vi "ReadTangoTestDoubleAttributes.vi"() -> ()   [LabVIEW 2009]
uses:
  tango_lv8/tango_vi.llb/ReadDoubleScalarAttribute.vi
  tango_lv8/tango_vi.llb/ReadDoubleSpectrumAttribute.vi
  tango_lv8/tango_vi.llb/ReadDoubleImageAttribute.vi
panel:
  out "Read/s":dbl
  out "Read/s":dbl
  in  "?":bool=TRUE
  in  "?":bool=TRUE
  out "Read/s":dbl
  in  "?":bool=TRUE
  out "error stack":string[](array[string])=["no error", "no error", "no error", "read_attributes"]
  out "error stack":string[](array[string])=["no error", "no error", "no error", "read_attributes"]
  out "error stack":string[](array[string])=["no error", "no error", "no error", "read_attributes"]
  out "scalar attr. value":dbl(graph)=99.87794428970838
  out "scalar attr. write value":dbl
  out "scalar attr. read value":dbl
  out "?":bool
  in  "attr_name":string="double_scalar"
  out "?":bool
  in  "attr_name":string="double_spectrum_ro"
  out "?":bool
  out "image attr. value":dbl[][](graph)
  out "spectrum attr. value":dbl[](graph)
  in  "attr_name":string="double_image_ro"
  in  "dev_name":string="tango/tangotest/1"
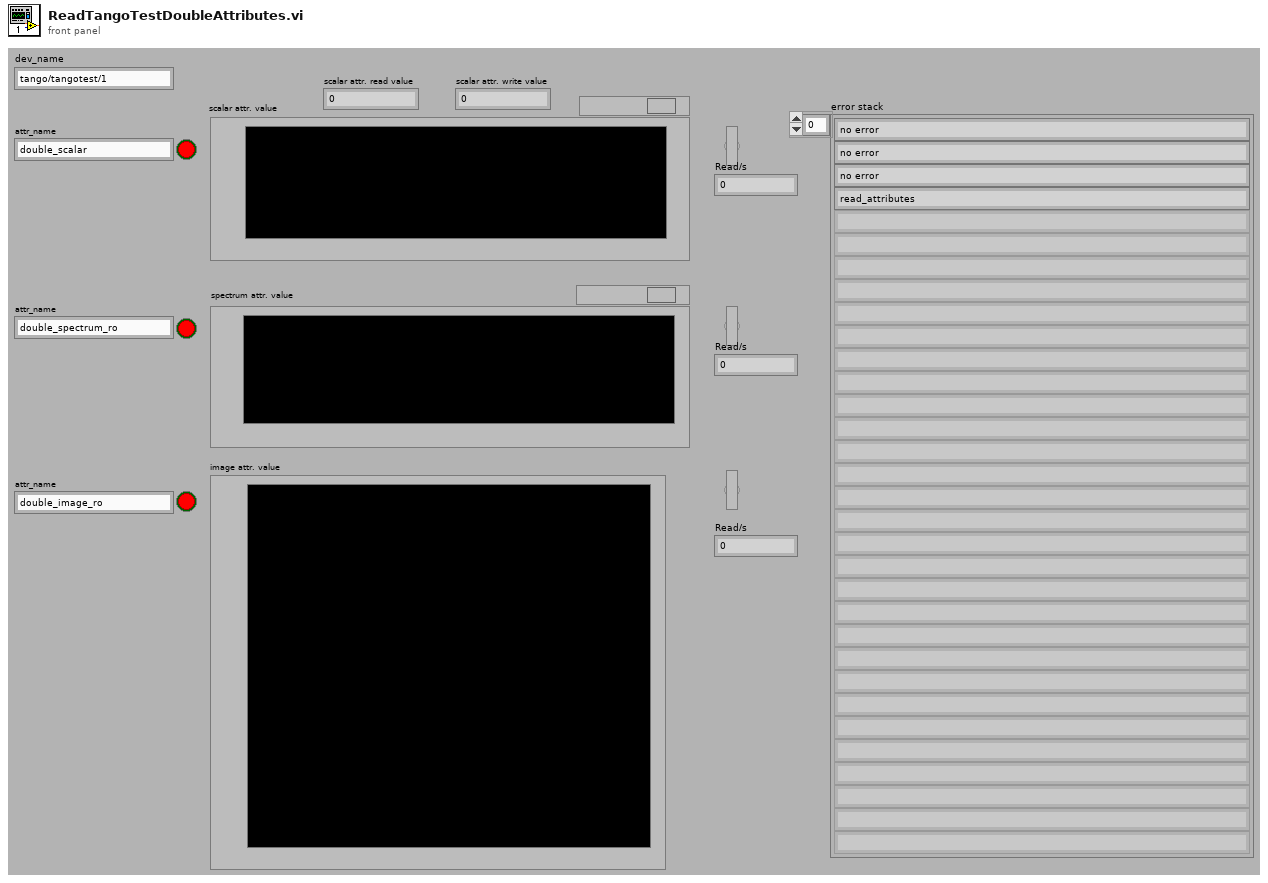
[diagram p1: front panel]
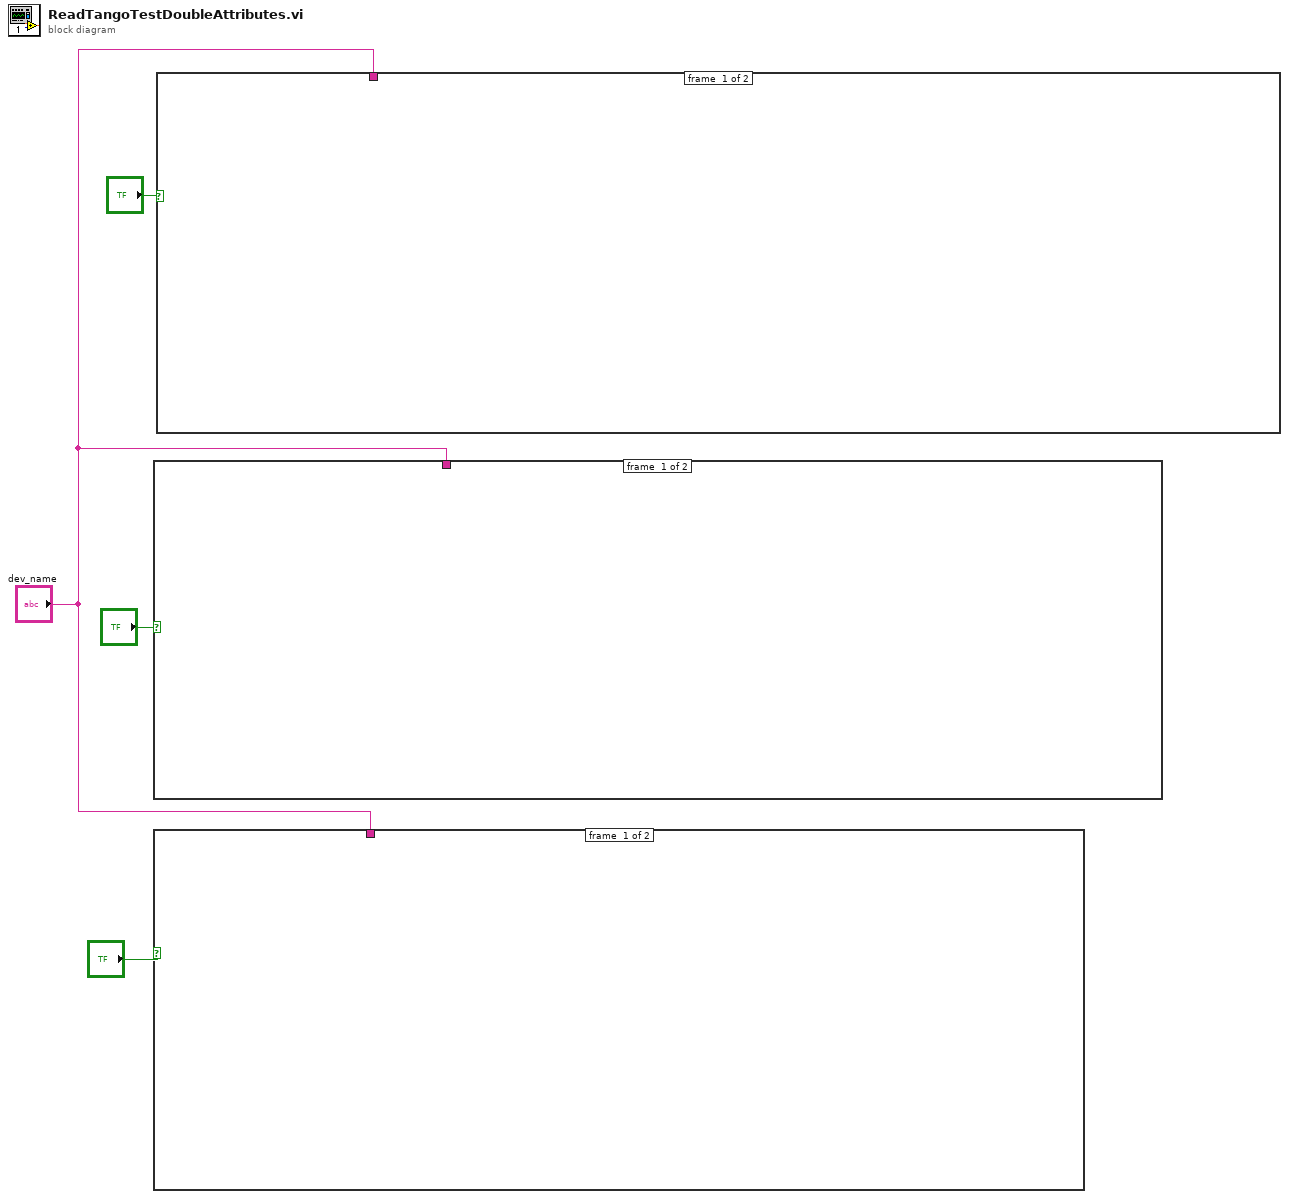
[diagram p0: block diagram]
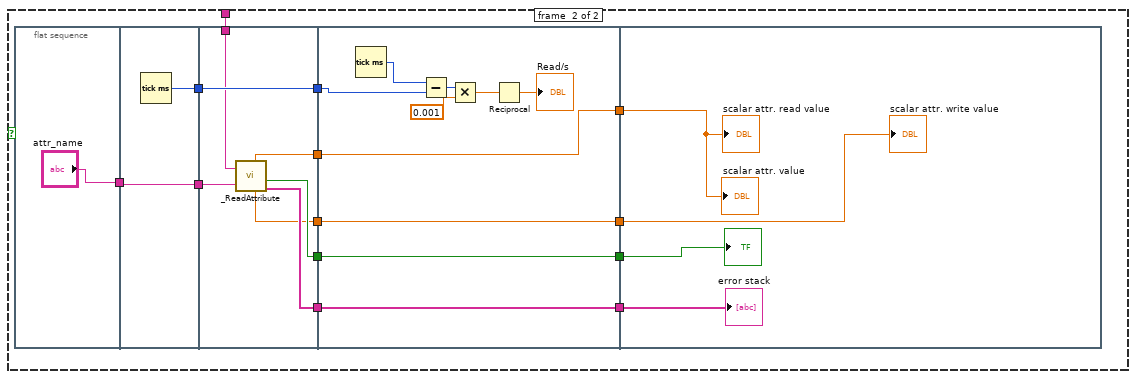
[diagram p2: hidden frame]
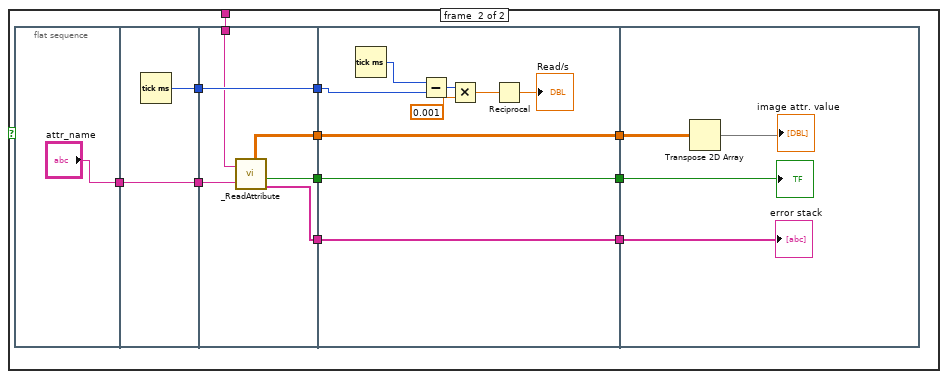
[diagram p3: hidden frame]
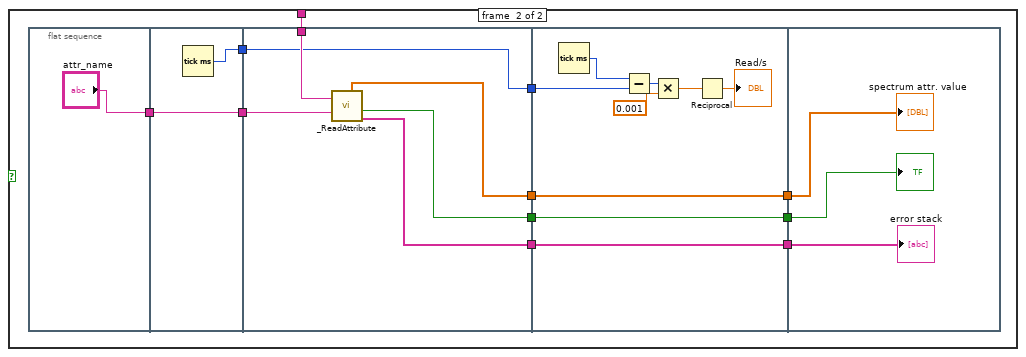
[diagram p4: hidden frame]
diagram:
  n1 = case shown="True" "?" {
    tunnel: "dev_name" -> [_ w9]
    frame #0 {
    }
    frame #1 {
      n2 = flat-sequence {
        tunnel: ["attr_name"] -> w15
        tunnel: [w18] -> w14
        tunnel: w15 -> [w18]
        tunnel: [w17] -> w13
        tunnel: w14 -> [w24]
        tunnel: w9 -> [w23]
        tunnel: w13 -> [w22]
        tunnel: [w21] -> w12
        tunnel: [w22] -> w11
        tunnel: [w19] -> w7
        tunnel: [w20] -> w5
        tunnel: [w31] -> w10
        tunnel: w12 -> [w31]
        tunnel: w11 -> [w28]
        tunnel: [w26] -> w8
        tunnel: w7 -> [w26]
        tunnel: [w25] -> w6
        tunnel: w5 -> [w25]
        tunnel: w10 -> [w36]
        tunnel: w8 -> [w35]
        tunnel: w6 -> [w34]
        frame #0 {
        }
        frame #1 {
          n3 = Tick Count (ms)() -> (millisecond timer value=w17:u32)
        }
        frame #2 {
          n4 = call-poly "_ReadAttribute.vi"("device name"=w23, "attribute name"=w24) -> ("value"=w21:dbl[], "success"=w19:bool, "error stack"=w20:string[])  [unwired: 3 out]
        }
        frame #3 {
          n5 = Tick Count (ms)() -> (millisecond timer value=w29:u32)
          n6 = Subtract(x=w29, y=w28) -> (x-y=w33:u32)
          n7 = Multiply(x=w33, y=0.001) -> (x*y=w30:dbl)
          n8 = Reciprocal(x=w30) -> (1/x=→"Read/s":dbl)
        }
        frame #4 {
          "?" <- w35
          "spectrum attr. value" <- w36
          "error stack" <- w34
        }
      }
    }
  }
  n9 = case shown="True" "?" {
    tunnel: "dev_name" -> [_ w43]
    frame #0 {
    }
    frame #1 {
      n10 = flat-sequence {
        tunnel: ["attr_name"] -> w46
        tunnel: [w50] -> w47
        tunnel: w46 -> [w50]
        tunnel: [w49] -> w45
        tunnel: w47 -> [w56]
        tunnel: w45 -> [w55]
        tunnel: [w55] -> w44
        tunnel: w43 -> [w54]
        tunnel: [w53] -> w41
        tunnel: [w52] -> w39
        tunnel: [w51] -> w37
        tunnel: w44 -> [w60]
        tunnel: [w59] -> w42
        tunnel: w41 -> [w59]
        tunnel: [w58] -> w40
        tunnel: w39 -> [w58]
        tunnel: [w57] -> w38
        tunnel: w37 -> [w57]
        tunnel: w42 -> [w68]
        tunnel: w40 -> [w67]
        tunnel: w38 -> [w66]
        frame #0 {
        }
        frame #1 {
          n11 = Tick Count (ms)() -> (millisecond timer value=w49:u32)
        }
        frame #2 {
          n12 = call-poly "_ReadAttribute.vi"("device name"=w54, "attribute name"=w56) -> ("value"=w53:dbl[][], "success"=w52:bool, "error stack"=w51:string[])  [unwired: 3 out]
        }
        frame #3 {
          n13 = Tick Count (ms)() -> (millisecond timer value=w61:u32)
          n14 = Subtract(x=w61, y=w60) -> (x-y=w65:u32)
          n15 = Multiply(x=w65, y=0.001) -> (x*y=w62:dbl)
          n16 = Reciprocal(x=w62) -> (1/x=→"Read/s":dbl)
        }
        frame #4 {
          n17 = Transpose 2D Array(2D array=w68) -> (transposed array=→"image attr. value":dbl[][])
          "?" <- w67
          "error stack" <- w66
        }
      }
    }
  }
  n18 = case shown="True" "?" {
    tunnel: "dev_name" -> [_ w79]
    frame #0 {
    }
    frame #1 {
      n19 = flat-sequence {
        tunnel: ["attr_name"] -> w80
        tunnel: [w85] -> w82
        tunnel: w80 -> [w84]
        tunnel: [w84] -> w72
        tunnel: w82 -> [w92]
        tunnel: [w92] -> w81
        tunnel: w79 -> [w88]
        tunnel: [w91] -> w77
        tunnel: [w90] -> w75
        tunnel: [w89] -> w73
        tunnel: w72 -> [w87]
        tunnel: [w86] -> w70
        tunnel: w81 -> [w97]
        tunnel: [w96] -> w78
        tunnel: w77 -> [w96]
        tunnel: [w95] -> w76
        tunnel: w75 -> [w95]
        tunnel: [w94] -> w74
        tunnel: w73 -> [w94]
        tunnel: [w93] -> w71
        tunnel: w70 -> [w93]
        tunnel: w78 -> [w104]
        tunnel: w76 -> [w106]
        tunnel: w74 -> [w105]
        tunnel: w71 -> [w103]
        frame #0 {
        }
        frame #1 {
          n20 = Tick Count (ms)() -> (millisecond timer value=w85:u32)
        }
        frame #2 {
          n21 = call-poly "_ReadAttribute.vi"("device name"=w88, "attribute name"=w87) -> ("value"=w91:dbl, "setpoint"=w86:dbl, "success"=w90:bool, "error stack"=w89:string[])  [unwired: 2 out]
        }
        frame #3 {
          n22 = Tick Count (ms)() -> (millisecond timer value=w98:u32)
          n23 = Subtract(x=w98, y=w97) -> (x-y=w102:u32)
          n24 = Multiply(x=w102, y=0.001) -> (x*y=w99:dbl)
          n25 = Reciprocal(x=w99) -> (1/x=→"Read/s":dbl)
        }
        frame #4 {
          "?" <- w106
          "scalar attr. read value" <- w104
          "scalar attr. value" <- w104
          "scalar attr. write value" <- w103
          "error stack" <- w105
        }
      }
    }
  }
